vi "test_simple_examples v0.vi"() -> ()   [LabVIEW 2018, in "LV-0mq-Julia_roundtrip-lib.lvlib"]
uses:
  LV-0mq-Julia_roundtrip-lib.lvlib
  Commands.ctl
  commands LV2Jl.ctl
  Server or client state.ctl
  d2cb43a9-9305-42fb-ad58-bce983510195.vi
  edf81fa3-46bf-427f-9605-85b461656974.vi
  <vilib>/measure/NI_MABase.lvlib
  9182218e-1e17-4e73-8c4b-7de0f475a335.vi
  35a44a82-786b-41ea-be73-9a4468e4df9d.vi
  StackFrame.ctl
  detailed error info.ctl
  simple examples functions.ctl
panel:
  out "Jl Server state":T1
  in  "execution control pages":enum32{"Start", "go - test", "finish"}(tab)
  in  "go":bool caption="go (Julia Server started externally)"
  in  "Start with Julia":bool caption="Start Julia Server and go"
  in  "p":dbl=1.0
  in  "fn":T2 caption="select function at Server" items=["arr_amplitude", "arr_length", "arr_mean", "arr_median", "arr_rms", "vec_amplify", "vec_attenuate", "vec_power"]
  in  "trim_at_begin":dbl
  in  "trim_at_end":dbl
  in  "Group":T3(tab)
  out "Server response":dbl
  out "data received plot":dbl[](graph)
  out "data received":dbl[](array[numeric]) format="%.3f"
  out "RMS":dbl
  out "detailed error info":T4
  out "current error":errorcluster
  out "final error":errorcluster
  out "short err code":u8
  in  "tones":T6(array[cluster])=[{"frequency"=10.0, "amplitude"=1.0, "phase"=0.0}, {"frequency"=20.0, "amplitude"=0.1, "phase"=0.0}] {"phase" format="%.2p"; "amplitude" format="%0.2p"; "frequency" format="%0.2p"}
  in  "noise (rms)":dbl=0.1 format="%.2p"
  in  "offset":dbl format="%.2p"
  in  "sampling info":cluster{"Fs":dbl, "#s":dbl}={"Fs"=1000.0, "#s"=1000.0} {"Fs" format="%.2p"}
  in  "next":bool
  out "data sent to server":dbl[](graph)
  out "data sent":dbl[](array[numeric]) format="%.3f"
  out "function name":string
  in  "stop both this VI and Julia Server":bool
  in  "stop this VI only":bool
  # "generate sample array"
  # "function and parameter"
  # "enter a negative or a large positive value to cause an exception"
  # "data returned by server"
  # "data sent to server"
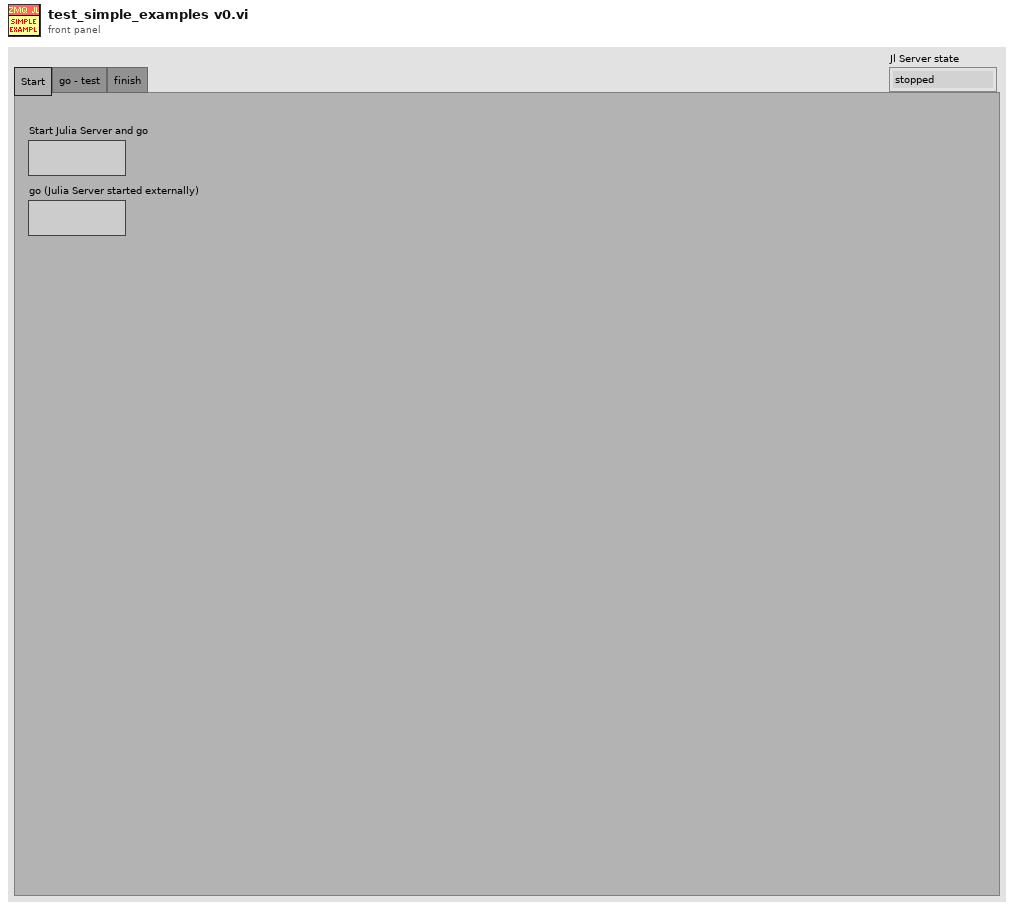
[diagram p1: front panel]
types:
  T1 = typedef "LV-0mq-Julia_roundtrip-lib.lvlib/Server or client state.ctl" = enum16{"stopped", "running", "unknown"}
  T2 = typedef "LV-0mq-Julia_roundtrip-lib.lvlib/simple examples functions.ctl" = u16
  T3 = enum32{"fns returning scalar", "fns returning vector", "error"}
  T4 = typedef "LV-0mq-Julia_roundtrip-lib.lvlib/detailed error info.ctl" = cluster{"exception_or_info":string, "trace":T5[]}
  T5 = typedef "LV-0mq-Julia_roundtrip-lib.lvlib/StackFrame.ctl" = cluster{"frame_summary":string, "func":string, "linfo":string, "file":string, "line":i32, "pointer":u64, "from_c":bool, "inlined":bool}
  T6 = cluster{"frequency":dbl, "amplitude":dbl, "phase":dbl}[]
  T7 = typedef "LV-0mq-Julia_roundtrip-lib.lvlib/Commands.ctl" = enum16{"Start Jl-server & Init LV-client", "Send request & Get response ", "Stop Jl-server & Cleanup LV-client", "Cleanup LV-client", "Start Jl-server", "Stop Jl-server", "Init LV-Client", "Cleanup LV-Client", "(not allowed)", "Set LV Client state", "Set Jl Server state", "set ZMQ timeout", "read ZMQ timeout", "read-out state"}
  T8 = enum8{"Enabled", "Disabled", "Disabled and Grayed Out"}
  T9 = typedef "LV-0mq-Julia_roundtrip-lib.lvlib/commands LV2Jl.ctl" = u8
  T10 = typedef "LV-0mq-Julia_roundtrip-lib.lvlib/Bindata&description.ctl" = cluster{"bindata_descr":T11[], "bindata":u8[]}
  T11 = typedef "LV-0mq-Julia_roundtrip-lib.lvlib/Bindata description.ctl" = cluster{"nofbytes":i32, "numtype":string, "start":i32, "arrdims":i32[], "kwarg_name":string, "category":string}
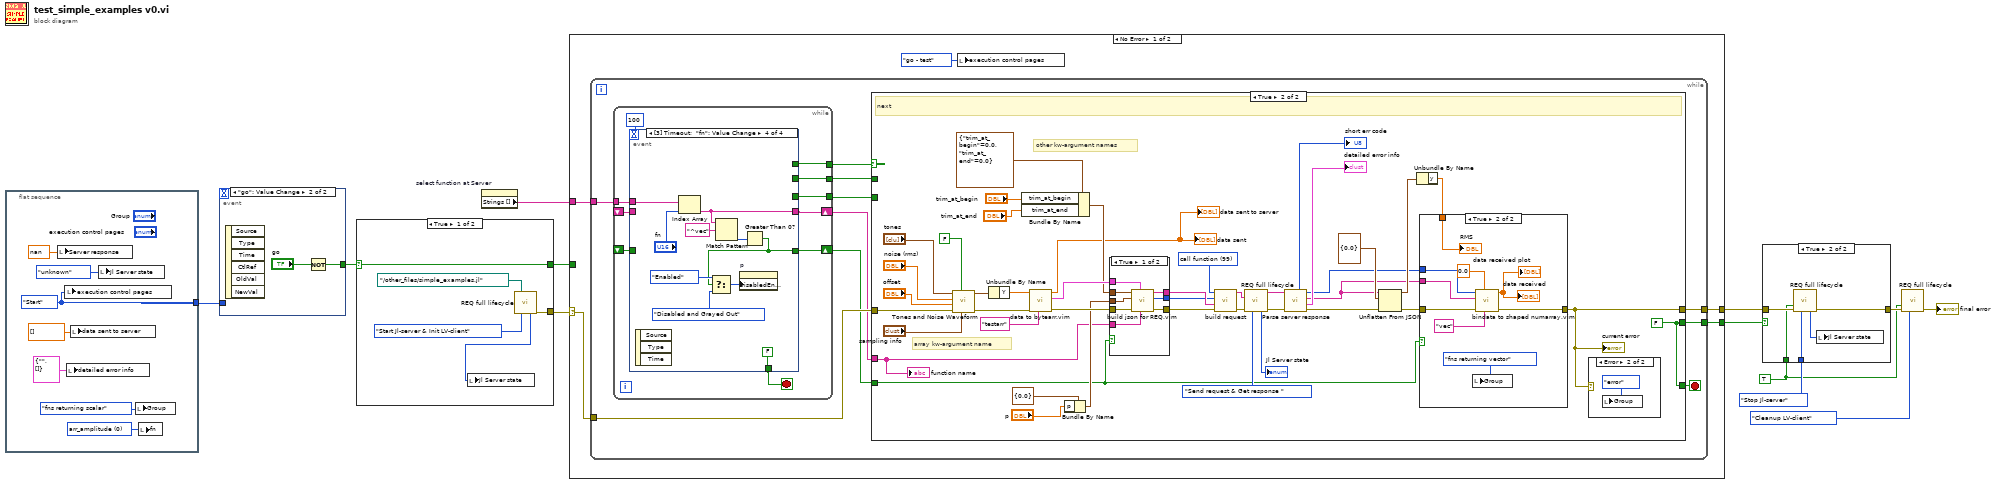
[diagram p0: block diagram]
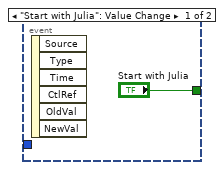
[diagram p2: hidden frame]
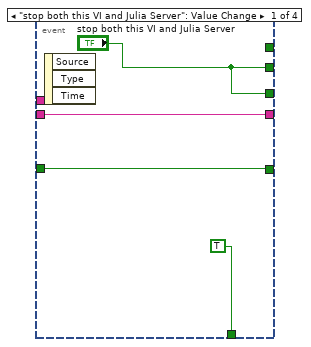
[diagram p3: hidden frame]
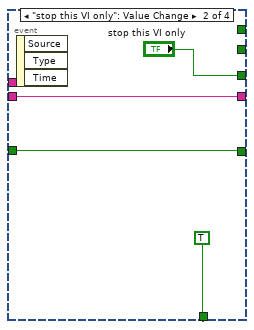
[diagram p4: hidden frame]
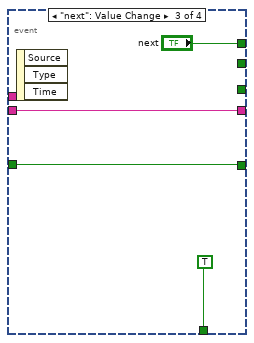
[diagram p5: hidden frame]
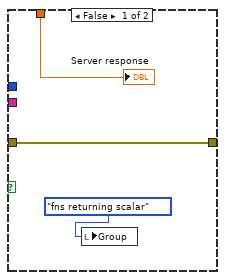
[diagram p7: hidden frame]
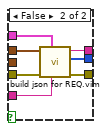
[diagram p8: hidden frame]
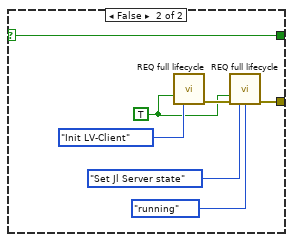
[diagram p11: hidden frame]
diagram:
  w7 = TRUE ("Force command")
  n1 = flat-sequence {
    tunnel: [w19] -> w1
    frame #0 {
      w13 = T2 0 items=["arr_amplitude", "arr_length", "arr_mean", "arr_median", "arr_rms", "vec_amplify", "vec_attenuate", "vec_power"] ("fn")
      w19 = enum32{"Start", "go - test", "finish"}."Start" ("execution control pages")
      n2 = local write "Server response"(nan ("Server response")) -> ()
      n3 = local write "execution control pages"(w19) -> ()
      n4 = local write "detailed error info"(T4 {"exception_or_info"="", "trace"=[]} ("detailed error info")) -> ()
      n5 = local write "data sent to server"(dbl[] []) -> ()
      n6 = local write "Jl Server state"(Server_or_client_state."unknown" ("Jl Server state out")) -> ()
      n7 = local write "Group"(T3."fns returning scalar" ("Group")) -> ()
      n8 = local write "fn"(w13) -> ()
    }
  }
  n9 = event shown="[1] \"go\": Value Change" {
    selector: _ -> [_ _]
    dyn-events: _ -> [_ _]
    timeout: _ -> [_ _]
    tunnel: ["Start with Julia" w21] -> w4
    tunnel: w1 -> [_ _]
    event "Start with Julia": Value Change {
      n10 = event-data() -> ()  [unwired: 1 in, 6 out]
    }
    event "go": Value Change {
      n11 = event-data() -> ()  [unwired: 1 in, 6 out]
      n12 = Not(x="go") -> (.not. x?=w21:bool)
    }
  }
  n13 = case shown="True" w4 {
    selector: w4 -> [w24 w28]
    tunnel: [w26 w29] -> w6
    tunnel: [w24 w28] -> w2
    frame True {
      n14 = call "REQ full lifecycle.vi"("Julia user functions script"=path "../other_files/simple_examples.jl", "command"=Commands."Start Jl-server & Init LV-client") -> ("Jl Server state out"=w23:T1, "error out"=w26:errorcluster)  [unwired: 7 in, 5 out]
      n15 = local write "Jl Server state"(w23) -> ()
    }
    frame False {
      w31 = TRUE ("Force command")
      n16 = call "REQ full lifecycle.vi"("Force command"=w31, "command"=Commands."Init LV-Client") -> ("error out"=w33:errorcluster)  [unwired: 7 in, 6 out]
      n17 = call "REQ full lifecycle.vi"("Force command"=w31, "error in"=w33, "command"=Commands."Set Jl Server state", "Jl Server state in"=Server_or_client_state."running") -> ("error out"=w29:errorcluster)  [unwired: 5 in, 6 out]
    }
  }
  n18 = property on="select function at Server" class="Ring (strict)"() -> ("Strings []"=w3:string[])  [unwired: 2 in, 2 out]
  n19 = case shown="No Error" w6 {
    selector: w6 -> [w38 w157]
    tunnel: [w39 w157] -> w12
    tunnel: [w37 w156] -> w5
    tunnel: w3 -> [w36 _]
    tunnel: w2 -> [_ w156]
    frame No Error {
      n20 = while {
        tunnel: w38 -> [w48]
        tunnel: [w49] -> w39
        tunnel: [w45] -> w37
        tunnel: w36 -> [w43]
        stop <- w46 stop-if-true
        n21 = while {
          tunnel: [w59] -> w47
          tunnel: [w58] -> w44
          tunnel: w43 -> [w55]
          shift-right: [w54] -> w42
          shift-left: _ -> [w51]
          shift-right: [w53] -> w41
          shift-left: _ -> [w52]
          tunnel: [w50] -> w40
          stop <- w57 stop-if-true
          n22 = event shown="[3] Timeout;  \"fn\": Value Change" {
            selector: _ -> [_ _ _ _]
            dyn-events: _ -> [_ _ _ _]
            timeout: 100 -> [_ _ _ _]
            tunnel: ["stop both this VI and Julia Server" _ _ _] -> w58
            tunnel: [_ _ "next" _] -> w59
            tunnel: [TRUE TRUE TRUE FALSE] -> w57
            tunnel: w55 -> [_ _ _ w75]
            tunnel: [w61 w65 w69 w74] -> w54
            tunnel: [w62 w66 w68 w73] -> w53
            tunnel: w52 -> [w62 w66 w68 _]
            tunnel: w51 -> [w61 w65 w69 _]
            tunnel: ["stop both this VI and Julia Server" "stop this VI only" _ _] -> w50
            event "stop both this VI and Julia Server": Value Change {
              n23 = event-data() -> ()  [unwired: 1 in, 3 out]
            }
            event "stop this VI only": Value Change {
              n24 = event-data() -> ()  [unwired: 1 in, 3 out]
            }
            event "next": Value Change {
              n25 = event-data() -> ()  [unwired: 1 in, 3 out]
            }
            event Timeout; Value Change {
              n26 = event-data() -> ()  [unwired: 1 in, 3 out]
              n27 = Index Array(array=w75, index="fn") -> (element=w73:string)
              n28 = Match Pattern(string=w73, regular expression="^vec") -> (offset past match=w79:i32)  [unwired: 1 in, 3 out]
              n29 = Greater Than 0?(x=w79) -> (x > 0?=w74:bool)
              n30 = Select(t=T8."Enabled" ("Disabled"), s=w74, f=T8."Disabled and Grayed Out" ("Disabled")) -> (s? t:f=w81:T8)
              n31 = property on="p" class="DigNum (strict)"("DisabledEnum"=w81) -> ()  [unwired: 2 in, 2 out]
            }
          }
        }
        n32 = case shown="True" w47 {
          tunnel: [w84 w91] -> w49
          tunnel: w48 -> [w84 w98]
          tunnel: [w83 w96] -> w46
          tunnel: w40 -> [w83 _]
          tunnel: [w82 w96] -> w45
          tunnel: w44 -> [w82 _]
          tunnel: w42 -> [_ w87]
          tunnel: w41 -> [_ w86]
          frame False {
            # "stop"
          }
          frame True {
            w96 = FALSE ("stop this VI only")
            w121 = T9 99 items=["call function"=99, "ping"=112, "stop"=115] ("Command")
            # "other kw-argument names"
            # "array kw-argument name"
            # "next"
            n33 = call <vilib>:"Tones and Noise Waveform.vi"("sampling info"="sampling info", "reset signal"=FALSE, "error in (no error)"=w98, "offset"="offset", "noise (rms)"="noise (rms)", "tones"="tones") -> ("error out"=w99:errorcluster, "signal out"=w105:waveform(dbl))  [unwired: 4 in]
            n34 = Unbundle By Name(w105) -> ("Y"=w100:dbl[])
            n35 = Bundle By Name(cluster=cluster{"trim_at_begin":dbl, "trim_at_end":dbl} {"trim_at_begin"=0.0, "trim_at_end"=0.0}, "trim_at_begin"="trim_at_begin", "trim_at_end"="trim_at_end") -> (w109:cluster{"trim_at_begin":dbl, "trim_at_end":dbl})
            n36 = call "data to bytearr.vim"("kwarg_name"="testarr", "error in (no error)"=w99, "data in"=w100) -> ("error out"=w112:errorcluster, "Bindata & descr out"=w113:T10, "flattened data out"=→"data sent" →"data sent to server":dbl[])  [unwired: 6 in]
            n37 = Bundle By Name(cluster=cluster{"p":dbl} {"p"=0.0}, "p"="p") -> (w95:cluster{"p":dbl})
            n38 = case shown="True" w87 {
              tunnel: [w147 w154] -> w126
              tunnel: [w146 w153] -> w118
              tunnel: [w145 w152] -> w117
              tunnel: w113 -> [w144 w151]
              tunnel: w112 -> [w143 w150]
              tunnel: w109 -> [w142 w149]
              tunnel: w86 -> [w141 w148]
              tunnel: w95 -> [w140 _]
              frame True {
                n39 = call "build json for REQ.vim"("fun2call"=w141, "Bindata & descr in"=w144, "error in (no error)"=w143, "Arguments 2"=w140, "Arguments 1"=w142) -> ("error out"=w147:errorcluster, "bindata out"=w145:u8[], "JSON string out"=w146:string)  [unwired: 4 in]
              }
              frame False {
                n40 = call "build json for REQ.vim"("fun2call"=w148, "Bindata & descr in"=w151, "error in (no error)"=w150, "Arguments 1"=w149) -> ("error out"=w154:errorcluster, "bindata out"=w152:u8[], "JSON string out"=w153:string)  [unwired: 5 in]
              }
            }
            n41 = call "build request.vi"("error in (no error)"=w126, "JSON data"=w118, "binary data"=w117, "Command"=w121) -> ("error out"=w124:errorcluster, "REQ string"=w125:string)  [unwired: 6 in]
            n42 = call "REQ full lifecycle.vi"("data to send"=w125, "error in"=w124, "command"=Commands."Send request & Get response ") -> ("server response"=w85:string, "Jl Server state out"=→"Jl Server state":T1, "error out"=w123:errorcluster)  [unwired: 6 in, 4 out]
            n43 = call "Parse server response.vi"("error in (no error)"=w123, "server response in"=w85) -> ("error out"=w116:errorcluster, "detailed error info"=→"detailed error info":T4, "JSON out"=w89:string, "binary data"=w90:u8[], "return code"=→"short err code":u8)  [unwired: 2 in, 3 out]
            n44 = Unflatten From JSON(JSON string=w89, type and defaults=cluster{"y":dbl} {"y"=0.0} ("parsed response"), error in (no error)=w116) -> (value=w114:cluster{"y":dbl}, error out=w92:errorcluster)  [unwired: 4 in]
            n45 = Unbundle By Name(w114) -> ("y"=w88:dbl)
            n46 = case shown="True" w87 {
              tunnel: w92 -> [w130 w138]
              tunnel: [w130 w137] -> w91
              tunnel: w90 -> [_ w136]
              tunnel: w89 -> [_ w135]
              tunnel: w88 -> [w128 w131]
              frame False {
                n47 = local write "Group"(T3."fns returning scalar" ("Group")) -> ()
                "Server response" <- w128
              }
              frame True {
                n48 = local write "Group"(T3."fns returning vector" ("Group")) -> ()
                n49 = call "bindata to shaped numarray.vim"("name"="vec" ("kwarg_name"), "data type"=0.0, "error in (no error)"=w138, "binary data"=w135, "JSON in"=w136) -> ("error out"=w137:errorcluster, "numarray 1D"=→"data received plot" →"data received":dbl[])  [unwired: 3 in, 2 out]
                "RMS" <- w131
              }
            }
            "current error" <- w91
            n50 = case shown="Error" w91 {
              frame No Error {
              }
              frame Error {
                n51 = local write "Group"(T3."error" ("Group")) -> ()
              }
            }
            "function name" <- w86
          }
        }
      }
      n52 = local write "execution control pages"(enum32{"Start", "go - test", "finish"}."go - test" ("execution control pages")) -> ()
    }
    frame Error {
    }
  }
  n53 = case shown="True" w5 {
    tunnel: w12 -> [w158 w163]
    tunnel: Commands."Stop Jl-server" ("command") -> [_ w162]
    tunnel: [w158 w161] -> w10
    tunnel: w7 -> [_ w160]
    frame False {
    }
    frame True {
      n54 = call "REQ full lifecycle.vi"("Force command"=w160, "error in"=w163, "command"=w162) -> ("Jl Server state out"=w159:T1, "error out"=w161:errorcluster)  [unwired: 6 in, 5 out]
      n55 = local write "Jl Server state"(w159) -> ()
    }
  }
  n56 = call "REQ full lifecycle.vi"("Force command"=w7, "error in"=w10, "command"=Commands."Cleanup LV-client") -> ("error out"=→"final error":errorcluster)  [unwired: 6 in, 6 out]
